vi "SPI_FREQ.vi"(1 "Device":enum16{"CAN", "ENC", "IMU1", "IMU2"}(ring)) -> (0 "Frequency (kHz)":u16=8000)   [LabVIEW 2019]
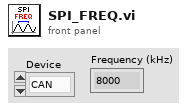
[diagram p1: front panel]
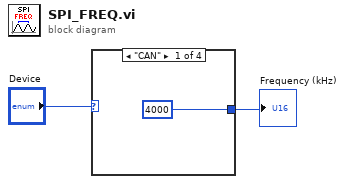
[diagram p0: block diagram]
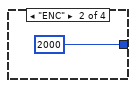
[diagram p2: hidden frame]
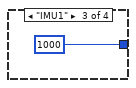
[diagram p3: hidden frame]
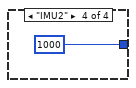
[diagram p4: hidden frame]
diagram:
  n1 = case shown="\"CAN\"" "Device" {
    tunnel: [u16 4000 u16 2000 u16 1000 u16 1000] -> w1
    frame "CAN" {
    }
    frame "ENC" {
    }
    frame "IMU1" {
    }
    frame "IMU2" {
    }
  }
  "Frequency (kHz)" <- w1
